vi "FileNameDuplicatedErrHandler.vi"(8 "Save Path (use dialog)":path=path "F:/Data/SUNYLymphNodeDB.txt", 11 "File Name":string) -> (0 "Save Path Out":path, 3 "File Name Out":string)   [LabVIEW 2022 SP3]
panel:
  in  "Done":bool
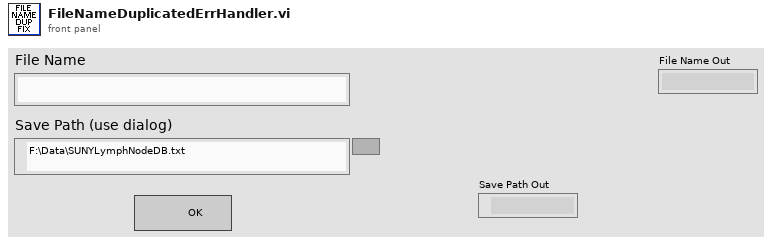
[diagram p1: front panel]
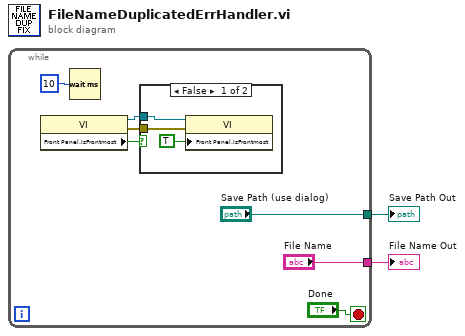
[diagram p0: block diagram]
diagram:
  n1 = while {
    tunnel: ["Save Path (use dialog)"] -> w2
    tunnel: ["File Name"] -> w1
    stop <- "Done" stop-if-true
    n2 = property class="VI"() -> (reference out=w4:refnum<vi>, error out=w6:errorcluster, "Front Panel.IsFrontmost"=w5:bool)  [unwired: 2 in]
    n3 = Wait (ms)(milliseconds to wait=u32 10) -> ()  [unwired: 1 out]
    n4 = case shown="False" w5 {
      tunnel: w4 -> [w12 _]
      tunnel: w6 -> [w10 _]
      frame False {
        n5 = property class="VI"(reference=w12, error in=w10, "Front Panel.IsFrontmost"=TRUE) -> ()  [unwired: 2 out]
      }
      frame True {
      }
    }
  }
  "File Name Out" <- w1
  "Save Path Out" <- w2
